vi "Create Folders.vi"(8 "error in (no error)":errorcluster, 11 "PostBuildSupport in":refnum<class "PostBuildSupport.lvclass">) -> (0 "error out":errorcluster, 3 "PostBuildSupport out":refnum<class "PostBuildSupport.lvclass">)   [LabVIEW 2016, in "PostBuildSupport.lvclass"]
uses:
  PostBuildSupport.lvclass
  PostBuildSupport.lvclass/PostBuildSupport.ctl
  <userlib>/_MGI/File/MGI Create Directory Chain Behavior Enum.ctl
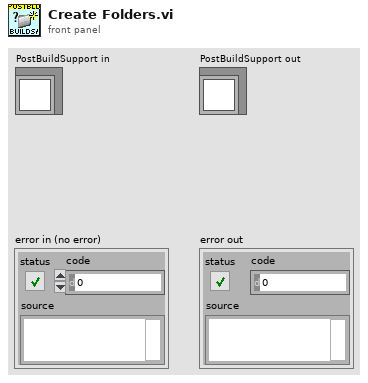
[diagram p1: front panel]
types:
  T1 = typedef "MGI Create Directory Chain Behavior Enum.ctl" = enum16{"Auto Detect", "Path Contains a File", "Path Does Not Contain a File"}
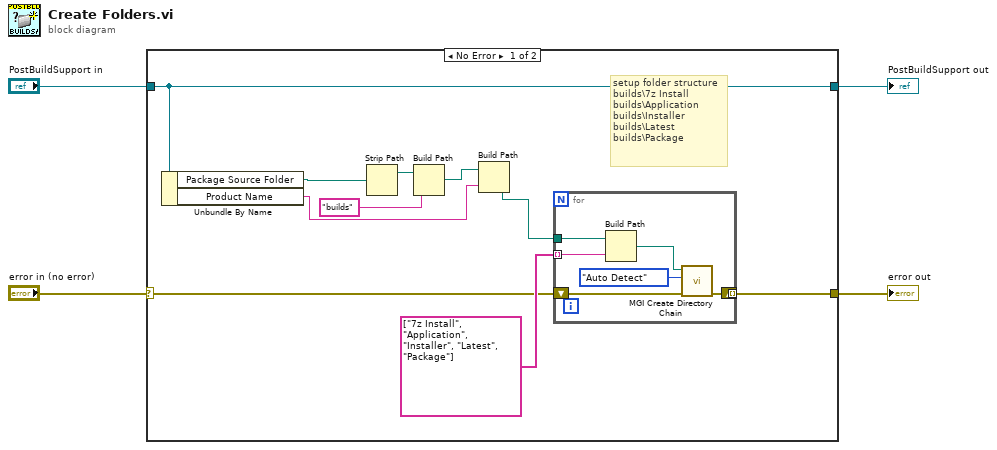
[diagram p0: block diagram]
diagram:
  n1 = case shown="No Error" "error in (no error)" {
    selector: "error in (no error)" -> [w6 w21]
    tunnel: "PostBuildSupport in" -> [w5 w22]
    tunnel: [w7 w21] -> w3
    tunnel: [w5 w22] -> w1
    frame No Error {
      # "setup folder structure\nbuilds\\7z Install\nbuilds\\Application\nbuilds\\Installer\nbuilds\\Latest\nbuilds\\Package"
      n2 = Unbundle By Name(w5) -> ("Package Source Folder"=w11:path, "Product Name"=w10:string)
      n3 = Strip Path(path=w11) -> (stripped path=w9:path)  [unwired: 1 out]
      n4 = Build Path(base path=w9, name or relative path="builds") -> (appended path=w12:path)
      n5 = Build Path(base path=w12, name or relative path=w10) -> (appended path=w8:path)
      n6 = for {
        shift-right: [w15] -> w7
        shift-left: w6 -> [w19]
        tunnel: w8 -> [w18]
        tunnel: string[] ["7z Install", "Application", "Installer", "Latest", "Package"] -> [w17] mode=indexing
        tunnel: [w15] -> _ mode=indexing
        n7 = Build Path(base path=w18, name or relative path=w17) -> (appended path=w16:path)
        n8 = call <userlib>:"MGI Create Directory Chain.vi"("Error In"=w19, "File Presence (Auto Detect)"=MGI_Create_Directory_Chain_Behavior_Enum."Auto Detect", "Path"=w16) -> ("Error Out"=w15:errorcluster)  [unwired: 7 in, 1 out]
      }
    }
    frame Error {
    }
  }
  "error out" <- w3
  "PostBuildSupport out" <- w1
